vi "Test Time Sync.vi"   [LabVIEW 2013]
uses:
  <vilib>/nisyscfg/nisyscfg.lvlib
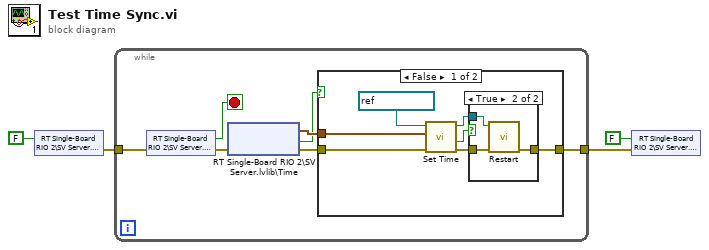
[diagram p0: block diagram]
diagram:
  n1 = shared-variable "RT Single-Board RIO 2\\SV Server.lvlib\\Stop"(FALSE ("Stop")) -> (error out=w2:errorcluster)  [unwired: 1 in]
  n2 = while {
    tunnel: [w5] -> w4
    tunnel: w2 -> [w10]
    stop <- w11 stop-if-true
    n3 = shared-variable "RT Single-Board RIO 2\\SV Server.lvlib\\Stop"(error in=w10) -> (w11:bool, error out=w7:errorcluster)
    n4 = shared-variable "RT Single-Board RIO 2\\SV Server.lvlib\\Time"(error in=w7) -> (w9:timestamp, error out=w6:errorcluster, w8:bool)  [unwired: 1 in]
    n5 = case shown="False" w8 {
      tunnel: w9 -> [w18 _]
      tunnel: w6 -> [w14 w23]
      tunnel: [w12 w23] -> w5
      frame False {
        n6 = call <vilib>:"Set Time.vi"("error in (no error)"=w14, "time"=w18, "session in (localhost)"=refnum<k21> "localhost") -> ("error out"=w13:errorcluster, "changes require restart"=w17:bool, "session out"=w16:refnum<k21>)  [unwired: 5 in, 1 out]
        n7 = case shown="True" w17 {
          tunnel: w16 -> [_ w22]
          tunnel: w13 -> [w19 w21]
          tunnel: [w19 w20] -> w12
          frame False {
          }
          frame True {
            n8 = call <vilib>:"Restart.vi"("error in (no error)"=w21, "session in"=w22) -> ("error out"=w20:errorcluster)  [unwired: 7 in, 2 out]
          }
        }
      }
      frame True {
      }
    }
  }
  n9 = shared-variable "RT Single-Board RIO 2\\SV Server.lvlib\\Stop"(FALSE ("Stop"), error in=w4) -> ()  [unwired: 1 out]
